vi "FREE_RECORD.vi"(8 "error in (no error)":errorcluster, 11 "Recordset Ref In":T2) -> (0 "error out":errorcluster, 3 "connection ref Out":T1)   [LabVIEW 2018, in "MySQLTools.lvlib"]
uses:
  MySQLTools.lvlib
  <vilib>/addons/database/Recordset.llb/Rec ObjectReference.ctl
  <vilib>/addons/database/Connection.llb/Conn ObjectReference.ctl
  <vilib>/addons/database/Recordset.llb/Rec Destroy - Connection.vi
  <vilib>/addons/database/NI_Database_API.lvlib
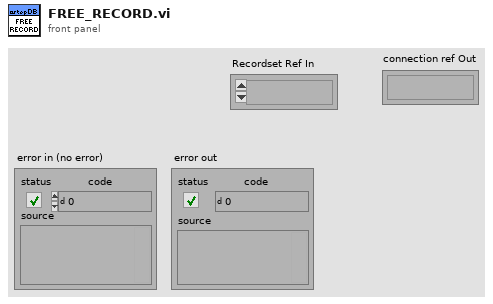
[diagram p1: front panel]
types:
  T1 = typedef "NI_Database_API.lvlib/Conn ObjectReference.ctl" = refnum<k1>
  T2 = typedef "NI_Database_API.lvlib/Rec ObjectReference.ctl" = refnum<k1>
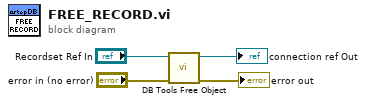
[diagram p0: block diagram]
diagram:
  n1 = call-poly <vilib>:"DB Tools Free Object.vi"("error in (no error)"="error in (no error)", "recordset reference"="Recordset Ref In") -> ("error out"=→"error out":errorcluster, "connection reference"=→"connection ref Out":T1)  [unwired: 8 in]
